vi "Initialization VI.vi"(8 "error in (no error)":errorcluster, 10 "Custom XML":string, 11 "Device Item Ref in":T1 format="%.0x") -> (0 "error out":errorcluster, 3 "Device Item Ref out":T1 format="%.0x")   [LabVIEW 2015, in "Import Export Sample Custom Device System Explorer.lvlib"]
uses:
  Import Export Sample Custom Device System Explorer.lvlib
  <vilib>/NI Veristand/Custom Device API/Custom Device Item Ref.ctl
  <vilib>/NI Veristand/Custom Device API/Custom Device Channel.ctl
  <vilib>/NI Veristand/Custom Device API/Custom Device Channel Type.ctl
  Shared/Constants.vi
  <vilib>/NI Veristand/Custom Device API/Set Item Property (String).vi
  <vilib>/NI/NIVS System Definition Utilities/System Definition Utilities.lvlib
  <vilib>/NI Veristand/Custom Device API/Custom Device API.lvlib
  Shared/Import Export Sample Custom Device Shared.lvlib
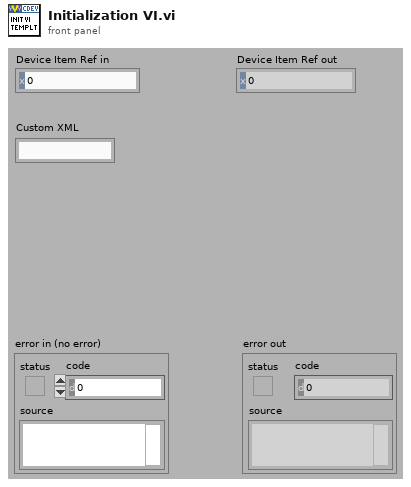
[diagram p1: front panel]
types:
  T1 = typedef "Custom Device API.lvlib/Custom Device Item Ref.ctl" = u64
  T2 = typedef "Custom Device API.lvlib/Custom Device Channel.ctl" = cluster{"Type":T3, "Units":string, "Default Value":dbl, "Faultable":bool, "Scalable":bool}
  T3 = typedef "Custom Device API.lvlib/Custom Device Channel Type.ctl" = enum16{"Input", "Output"}
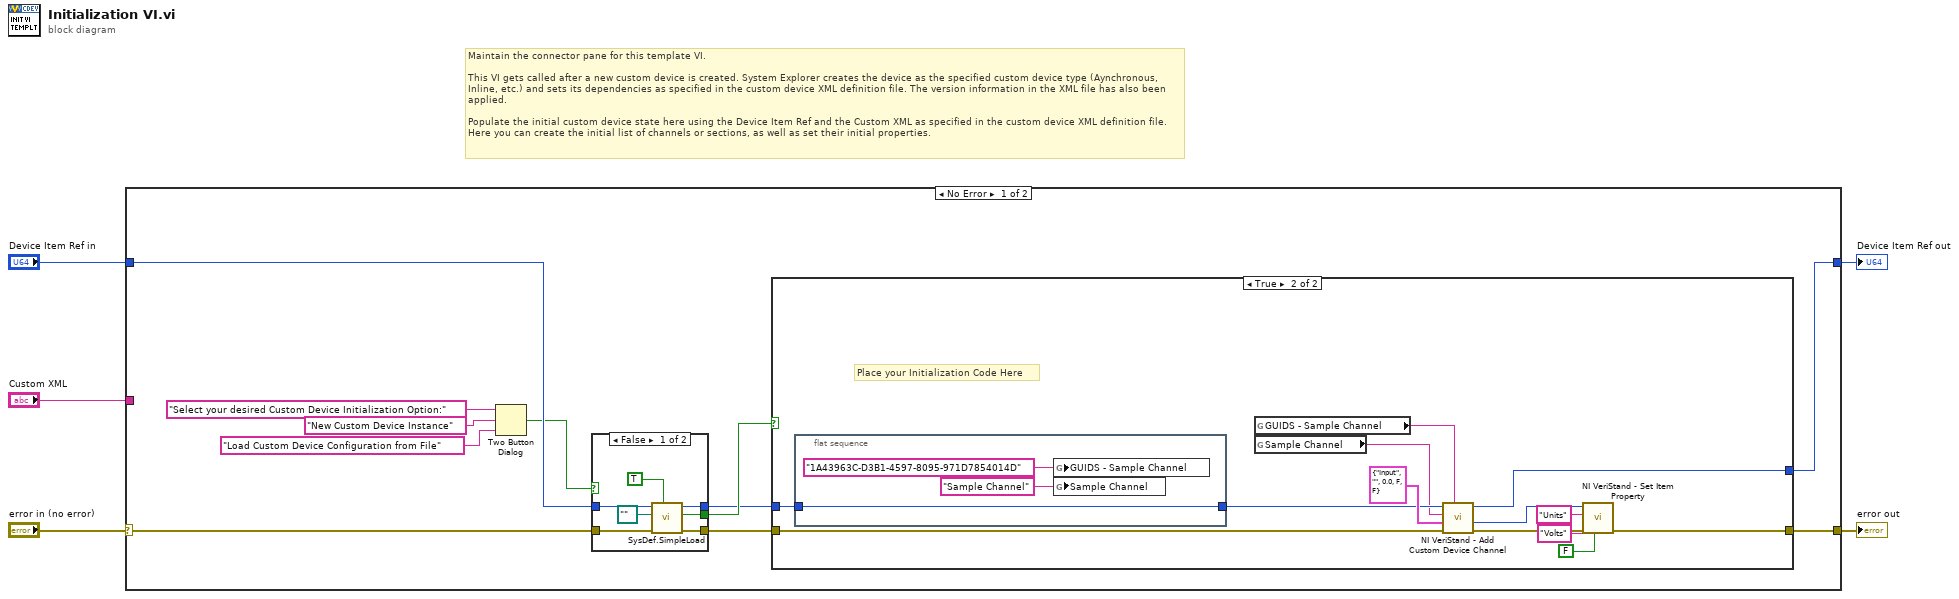
[diagram p0: block diagram]
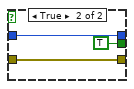
[diagram p2: hidden frame]
diagram:
  # "Maintain the connector pane for this template VI.\n\nThis VI gets called after a new custom device is created. System Explorer creates the device as the specified custom device type (Aynchronous, Inline, etc.) and sets its dependencies as specified in the custom device XML definition file. The version information in the XML file has also been applied.\n\nPopulate the initial custom device state here using the Device Item Ref and the Custom XML as specified in the custom device XML definition file. Here you can create the initial list of channels or sections, as well as set their initial properties."
  n1 = case shown="No Error" "error in (no error)" {
    selector: "error in (no error)" -> [w10 w46]
    tunnel: [w13 w46] -> w5
    tunnel: [w12 w45] -> w3
    tunnel: "Device Item Ref in" -> [w11 w45]
    tunnel: "Custom XML" -> [_ _]
    frame No Error {
      n2 = Two Button Dialog(message="Select your desired Custom Device Initialization Option:", 1:"Load Custom Device Configuration from File" ("F button name (\"Cancel\")"), 2:"New Custom Device Instance" ("T button name (\"OK\")")) -> (T button?=w9:bool)
      n3 = case shown="False" w9 {
        tunnel: w11 -> [w21 w24]
        tunnel: w10 -> [w20 w26]
        tunnel: [w19 w26] -> w8
        tunnel: [w18 TRUE ("cancelled")] -> w7
        tunnel: [w17 w24] -> w6
        frame False {
          n4 = call <vilib>:"SysDef.SimpleLoad.vi"("Overwrite Existing?"=TRUE, "error in (no error)"=w20, "Path"=path "", "NodeID"=w21) -> ("error out"=w19:errorcluster, "cancelled"=w18:bool, "NodeID out"=w17:u64)  [unwired: 5 in]
        }
        frame True {
        }
      }
      n5 = case shown="True" w7 {
        tunnel: w8 -> [w27 w39]
        tunnel: [w27 w36] -> w13
        tunnel: w6 -> [w28 w32]
        tunnel: [w28 w33] -> w12
        frame False {
        }
        frame True {
          # "Place your Initialization Code Here"
          n6 = flat-sequence {
            tunnel: w32 -> [w42]
            tunnel: [w42] -> w31
            frame #0 {
              n7 = global write "Constants.vi" "GUIDS - Sample Channel"("1A43963C-D3B1-4597-8095-971D7854014D" ("GUIDS - Sample Channel")) -> ()
              n8 = global write "Constants.vi" "Sample Channel"("Sample Channel" ("Sample Channel")) -> ()
            }
          }
          n9 = global read "Constants.vi" "GUIDS - Sample Channel"() -> (w30:string)
          n10 = global read "Constants.vi" "Sample Channel"() -> (w29:string)
          n11 = call <vilib>:"NI VeriStand - Add Custom Device Channel.vi"("GUID (Default Channel)"=w30, "error in (no error)"=w39, "Channel"=T2 {"Type"=enum."Input", "Units"="", "Default Value"=0.0, "Faultable"=FALSE, "Scalable"=FALSE}, "Channel Name"=w29, "Parent Ref in"=w31) -> ("error out"=w40:errorcluster, "Channel Ref"=w35:T1, "Parent Ref out"=w33:T1)  [unwired: 3 in, 1 out]
          n12 = call-poly <vilib>:"NI VeriStand - Set Item Property.vi"("Binary String (T)"=FALSE, "error in (no error)"=w40, "Value"="Volts", "Property Name"="Units", "Item Ref in"=w35) -> ("error out"=w36:errorcluster)  [unwired: 4 in, 2 out]
        }
      }
    }
    frame Error {
    }
  }
  "error out" <- w5
  "Device Item Ref out" <- w3
